vi "Acquisizione statica_1.vi"() -> ()   [LabVIEW 2017]
uses:
  <vilib>/Analysis/4window.llb/windowTd.ctl
  <vilib>/measure/maspectr.llb/Power Spectrum and PSD Export Mode.ctl
  <vilib>/DAQmx/read.llb/DAQmx Read (Analog 1D Wfm NChan NSamp).vi
  <vilib>/DAQmx/configure/timing.llb/DAQmx Timing (Sample Clock).vi
  <vilib>/DAQmx/miscellaneous.llb/DAQmx Fill In Error Info.vi
  <vilib>/measure/maspectr.llb/FFT Power Spectrum and PSD for N Chan.vi
  <vilib>/measure/maspectr.llb/FFT Spectrum (Mag-Phase) for N Chan.vi
  <vilib>/measure/maspectr.llb/Frequency Response Function (Mag-Phase) N-M.vi
  <vilib>/Waveform/WDTOps.llb/WDT Index Channel DBL.vi
  <vilib>/Waveform/WDTOps.llb/WDT Append Waveforms DBL.vi
  <vilib>/measure/NI_MAPro.lvlib
  <vilib>/Analysis/NI_AALPro.lvlib
panel:
  in  "temperatura":refnum<k21>
  out "Massa pesata":string
  out "iterazioni":i32
  out "errore":bool
  out "error out":errorcluster
  out "std dev":bool
  out "mean":bool
  out "sample":i32
  in  "std dev max":dbl=6e-07
  in  "mean/sample max":dbl=0.002
  out "mean/sample":dbl
  out "mean":dbl format="%0.2f"
  out "std dev/semple":dbl
  out "standard deviation":dbl format="%0.2f"
  in  "Massa":string="_"
  in  "secondi da salvare":i32=30
  in  "restart averaging (F)":bool
  in  "window":T1 items=["Rectangle"=0, "Hanning"=1, "Hamming"=2, "Blackman-Harris"=3, "Exact Blackman"=4, "Blackman"=5, "Flat Top"=6, "4 Term B-Harris "=7, "7 Term B-Harris"=8, "Low Sidelobe"=9, "Blackman Nuttall"=11, "Triangle"=30, "Bartlett-Hanning"=31, "Bohman"=32, "Parzen"=33, "Welch"=34, "Kaiser"=60, "Dolph-Chebyshev"=61, "Gaussian"=62]
  in  "averaging parameters":T2={"averaging mode"=enum."Vector averaging", "weighting mode"=enum."Linear", "number of averages"=1000}
  in  "Tab Control 2":enum32{"LC", "T", "FRF", "PSD", "FFT"}(tab)
  out "Load Cell":waveform(dbl)[](graph)
  out "Temperature":waveform(dbl)[](graph)
  out "Waveform Graph":cluster{"f0":dbl, "df":dbl, "magnitude":dbl[]}[](graph)
  out "Waveform Graph 2":cluster{"f0":dbl, "df":dbl, "magnitude":dbl[]}[](graph)
  out "Magnitude 2":cluster{"f0":dbl, "df":dbl, "magnitude":dbl[]}[](graph)
  out "Magnitude":cluster{"f0":dbl, "df":dbl, "magnitude":dbl[]}[](graph)
  in  "SAVE?":bool
  in  "export":path
  in  "stop":bool
  in  "acquisition":T3={"Fs"=2000.0, "group sample/s"=10, "generation task"="ModAnalEs"} {"Fs" format="%.2p"}
  # "0,002"
  # "x10^-3"
  # "x10^-6"
  # "6E-7"
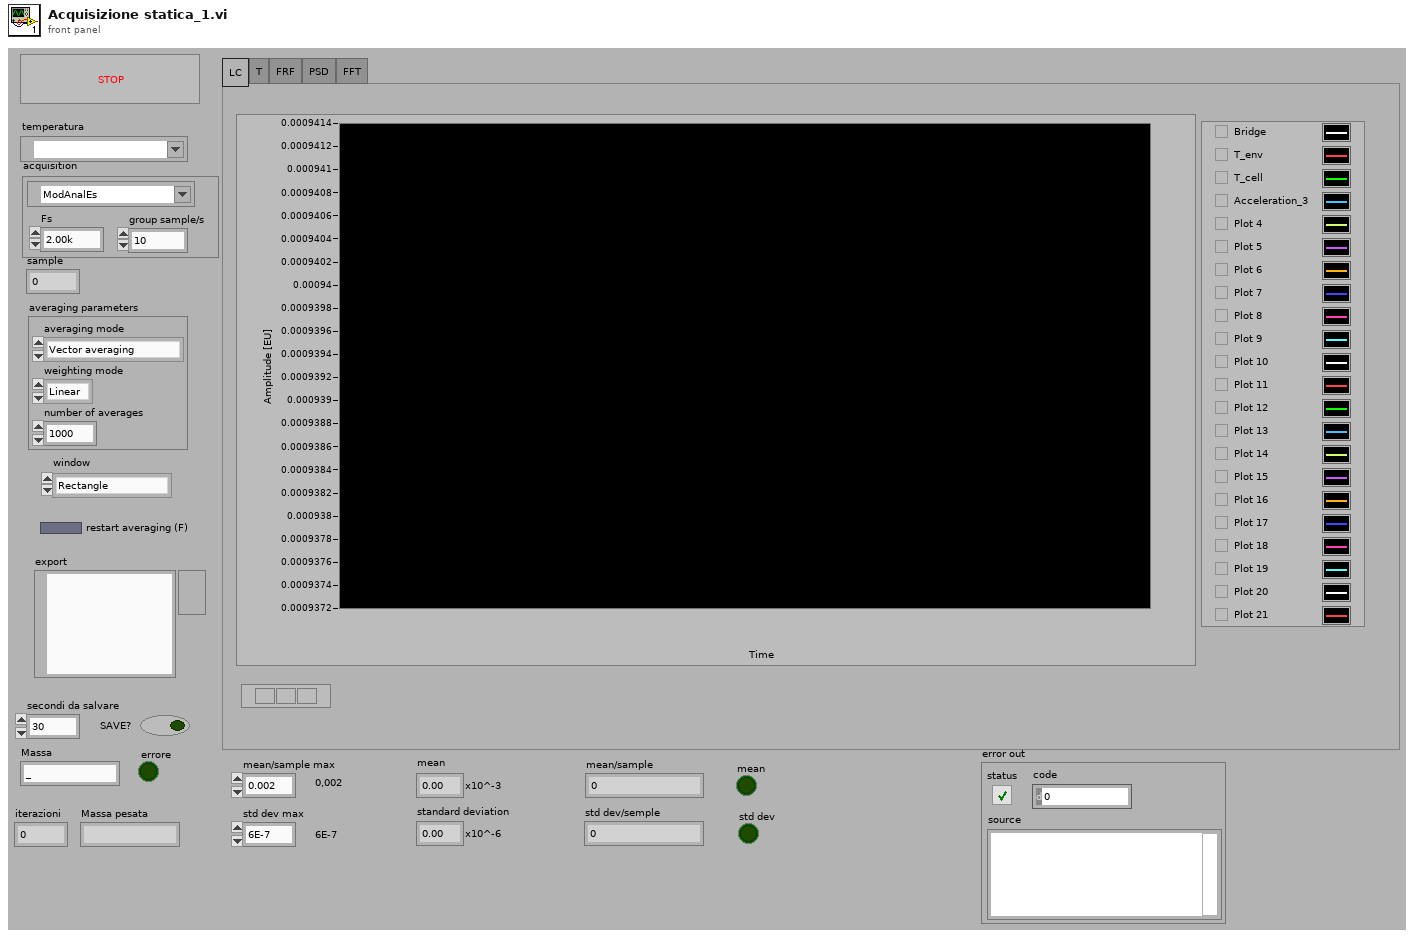
[diagram p1: front panel]
types:
  T1 = typedef "NI_AALPro.lvlib/windowTd.ctl" = u32
  T2 = cluster{"averaging mode":enum16{"No averaging", "Vector averaging", "RMS averaging", "Peak hold"}, "weighting mode":enum16{"Linear", "Exponential"}, "number of averages":u32}
  T3 = cluster{"Fs":dbl, "group sample/s":i32, "generation task":refnum<k21>}
  T4 = cluster{"dB On (F)":bool, "unwrap phase (F)":bool, "convert to degree (F)":bool}
  T5 = typedef "NI_MAPro.lvlib/Power Spectrum and PSD Export Mode.ctl" = u16
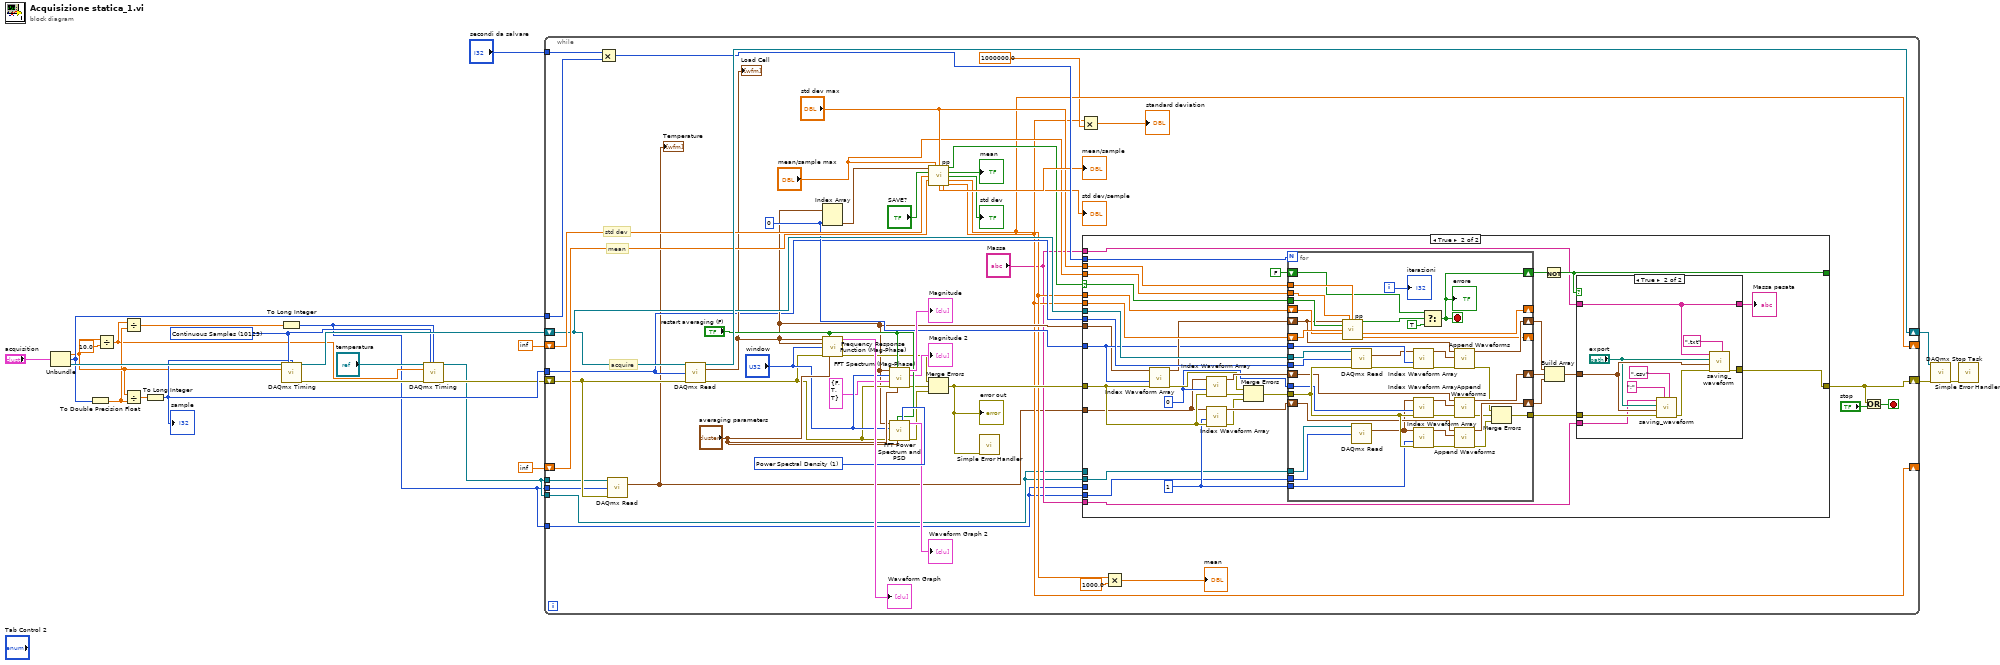
[diagram p0: block diagram]
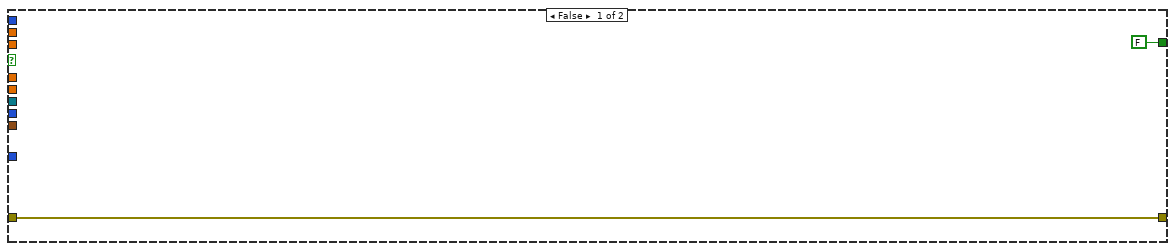
[diagram p2: hidden frame]
diagram:
  w11 = 10123 items=["Finite Samples"=10178, "Continuous Samples"=10123, "Hardware Timed Single Point"=12522] ("sample mode")
  n1 = Unbundle("acquisition") -> ("Fs"=w9:dbl, "group sample/s"=w13:i32, "generation task"=w20:refnum<k21>)
  n2 = To Double Precision Float(number=w13) -> (double precision float=w7:dbl)
  n3 = Divide(x=w9, y=10.0) -> (x/y=w3:dbl)
  n4 = Divide(x=w3, y=w7) -> (x/y=w6:dbl)
  n5 = Divide(x=w9, y=w7) -> (x/y=w16:dbl)
  n6 = To Long Integer(number=w16) -> (32bit integer=w10:i32)
  "sample" <- w10
  n7 = To Long Integer(number=w6) -> (32bit integer=w1:i32)
  n8 = call-poly <vilib>:"DAQmx Timing.vi"("task/channels in"=w20, "sample mode"=w11, "samples per channel"=w10, "rate"=w9) -> ("task out"=w19:refnum<k21>, "error out"=w5:errorcluster)  [unwired: 10 in]
  n9 = call-poly <vilib>:"DAQmx Timing.vi"("task/channels in"="temperatura", "sample mode"=w11, "samples per channel"=w1, "rate"=w3, "error in"=w5) -> ("task out"=w2:refnum<k21>, "error out"=w4:errorcluster)  [unwired: 9 in]
  n10 = while {
    shift-right: [w72] -> w22
    shift-left: w19 -> [w57]
    shift-right: [w60] -> w23
    shift-left: w4 -> [w29]
    tunnel: w13 -> [w56]
    shift-right: [w36] -> _
    shift-left: inf -> [w59]
    shift-right: [w32] -> _
    shift-left: inf -> [w58]
    tunnel: "secondi da salvare" -> [w54]
    tunnel: w10 -> [w37]
    tunnel: w2 -> [w27]
    tunnel: w1 -> [w28]
    tunnel: w2 -> [w25]
    tunnel: w1 -> [w24]
    stop <- w61 stop-if-true
    w40 = 0 ("REFERENCE CHANNEL")
    w70 = T5 1 items=["Power Spectrum", "Power Spectral Density"] ("export mode")
    # "mean"
    # "std dev"
    # "acquire"
    n11 = Multiply(x=w54, y=w56) -> (x*y=w55:i32)
    n12 = call-poly <vilib>:"DAQmx Read.vi"("task/channels in"=w27, "number of samples per channel"=w28, "error in"=w29) -> ("data"=w26:waveform(dbl)[])  [unwired: 10 in, 2 out]
    "Temperature" <- w26
    n13 = call-poly <vilib>:"DAQmx Read.vi"("task/channels in"=w57, "number of samples per channel"=w37, "error in"=w29) -> ("task out"=w72:refnum<k21>, "data"=w38:waveform(dbl)[], "error out"=w44:errorcluster)  [unwired: 10 in]
    "Load Cell" <- w38
    n14 = Index Array(array=w38, index #2=w40) -> (element #2=w53:waveform(dbl))  [unwired: 1 in, 1 out]
    n15 = call-poly <vilib>:"Frequency Response Function (Mag-Phase).vi"("time signals X"=w38, "restart averaging (F)"="restart averaging (F)", "time signals Y"=w38, "window"="window", "error in (no error)"=w44, "averaging parameters"="averaging parameters") -> ("magnitudes"=→"Waveform Graph":cluster{"f0":dbl, "df":dbl, "magnitude":dbl[]}[], "error out"=w41:errorcluster)  [unwired: 4 in, 4 out]
    n16 = call-poly <vilib>:"FFT Spectrum (Mag-Phase).vi"("averaging parameters"="averaging parameters", "restart averaging (F)"="restart averaging (F)", "error in (no error)"=w44, "view"=T4 {"dB On (F)"=FALSE, "unwrap phase (F)"=TRUE, "convert to degree (F)"=TRUE}, "window"="window", "time signals"=w38) -> ("error out"=w42:errorcluster, "phases"=→"Magnitude 2":cluster{"f0":dbl, "df":dbl, "phase":dbl[]}[], "magnitudes"=→"Magnitude":cluster{"f0":dbl, "df":dbl, "magnitude":dbl[]}[])  [unwired: 1 in, 2 out]
    n17 = call-poly <vilib>:"FFT Power Spectrum and PSD.vi"("export mode"=w70, "averaging parameters"="averaging parameters", "restart averaging (F)"="restart averaging (F)", "error in (no error)"=w44, "window"="window", "time signals"=w38) -> ("error out"=w43:errorcluster, "Power Spectrum / PSD"=→"Waveform Graph 2":cluster{"f0":dbl, "df":dbl, "magnitude":dbl[]}[])  [unwired: 2 in, 2 out]
    n18 = call "pp.vi"("Waveform"=w53, "mean/sample max"="mean/sample max", "std dev max"="std dev max", "SAVE?"="SAVE?", "prev std dev"=w59, "prev mean"=w58) -> ("out"=w49:bool, 6:"mean"=→"mean":bool, "std dev"=→"std dev":bool, 10:"mean"=w36:dbl, "std dev/semple"=→"std dev/semple":dbl, "mean/sample"=→"mean/sample":dbl, "standard deviation"=w32:dbl)  [unwired: 3 in]
    n19 = Merge Errors(w41, w42, w43) -> (w39:errorcluster)
    "error out" <- w39
    n20 = call <vilib>:"Simple Error Handler.vi"("error in (no error)"=w39) -> ()  [unwired: 4 in, 5 out]
    n21 = Multiply(x=w32, y=1000000.0) -> (x*y=→"standard deviation":dbl)
    n22 = case shown="True" w49 {
      selector: w49 -> [_ w102]
      tunnel: w39 -> [w74 w87]
      tunnel: [w74 w109] -> w60
      tunnel: w38 -> [_ w82]
      tunnel: w55 -> [_ w108]
      tunnel: w57 -> [_ w107]
      tunnel: w37 -> [_ w105]
      tunnel: w32 -> [_ w101]
      tunnel: w36 -> [_ w100]
      tunnel: "std dev max" -> [_ w99]
      tunnel: "mean/sample max" -> [_ w98]
      tunnel: [FALSE w95] -> _
      tunnel: w40 -> [_ w93]
      tunnel: "Massa" -> [_ w92]
      tunnel: "Massa" -> [_ w91]
      tunnel: w25 -> [_ _]
      tunnel: w24 -> [_ _]
      tunnel: w26 -> [_ w77]
      tunnel: w25 -> [_ w76]
      tunnel: w24 -> [_ w75]
      frame False {
      }
      frame True {
        w80 = 1 ("index")
        w81 = 0 ("index")
        n23 = call-poly <vilib>:"Index Waveform Array.vi"("error in (no error)"=w87, "index"=w93, "waveform array"=w82) -> ("error out"=w86:errorcluster, "waveform"=w94:waveform(dbl))  [unwired: 7 in]
        n24 = call-poly <vilib>:"Index Waveform Array.vi"("error in (no error)"=w87, "index"=w81, "waveform array"=w77) -> ("error out"=w85:errorcluster, "waveform"=w89:waveform(dbl))  [unwired: 7 in]
        n25 = call-poly <vilib>:"Index Waveform Array.vi"("error in (no error)"=w87, "index"=w80, "waveform array"=w77) -> ("error out"=w84:errorcluster, "waveform"=w88:waveform(dbl))  [unwired: 7 in]
        n26 = Merge Errors(w86, w85, w84) -> (w83:errorcluster)
        n27 = for {
          N: w108 -> [_]
          shift-right: [w148] -> w104
          shift-left: w94 -> [w131]
          tunnel: [w115] -> w106
          tunnel: w83 -> [w128]
          tunnel: w107 -> [w144]
          tunnel: w105 -> [w143]
          tunnel: w102 -> [w142]
          shift-right: [w138] -> _
          shift-left: w101 -> [w141]
          shift-right: [w139] -> _
          shift-left: w100 -> [w140]
          tunnel: w99 -> [w137]
          tunnel: w98 -> [w136]
          shift-right: [w129] -> w96
          shift-left: FALSE -> [w134]
          tunnel: w93 -> [w132]
          shift-right: [w124] -> w79
          shift-left: w89 -> [w126]
          shift-right: [w121] -> w78
          shift-left: w88 -> [w122]
          tunnel: w81 -> [w127]
          tunnel: w80 -> [w113]
          tunnel: w76 -> [w112]
          tunnel: w75 -> [w111]
          i -> [w130]
          stop <- w129 stop-if-true
          n28 = call "pp.vi"("Waveform"=w131, "mean/sample max"=w136, "std dev max"=w137, "SAVE?"=w142, "prev std dev"=w141, "prev mean"=w140) -> ("out"=w135:bool, "mean"=w139:dbl, "standard deviation"=w138:dbl)  [unwired: 3 in, 4 out]
          n29 = call-poly <vilib>:"DAQmx Read.vi"("task/channels in"=w144, "number of samples per channel"=w143, "error in"=w128) -> ("data"=w114:waveform(dbl)[], "error out"=w146:errorcluster)  [unwired: 10 in, 1 out]
          n30 = call-poly <vilib>:"DAQmx Read.vi"("task/channels in"=w112, "number of samples per channel"=w111) -> ("data"=w110:waveform(dbl)[])  [unwired: 11 in, 2 out]
          n31 = call-poly <vilib>:"Index Waveform Array.vi"("error in (no error)"=w146, "index"=w132, "waveform array"=w114) -> ("error out"=w145:errorcluster, "waveform"=w147:waveform(dbl))  [unwired: 7 in]
          n32 = call-poly <vilib>:"Index Waveform Array.vi"("error in (no error)"=w128, "index"=w127, "waveform array"=w110) -> ("error out"=w119:errorcluster, "waveform"=w125:waveform(dbl))  [unwired: 7 in]
          n33 = call-poly <vilib>:"Index Waveform Array.vi"("error in (no error)"=w128, "index"=w113, "waveform array"=w110) -> ("error out"=w120:errorcluster, "waveform"=w123:waveform(dbl))  [unwired: 7 in]
          n34 = Select(t=w134, s=w135, f=TRUE) -> (s? t:f=w129:bool)
          "errore" <- w129
          n35 = call-poly <vilib>:"Append Waveforms.vi"("error in (no error)"=w145, "waveform B"=w147, "waveform A"=w131) -> ("error out"=w116:errorcluster, "waveform out"=w148:waveform(dbl))  [unwired: 7 in]
          n36 = call-poly <vilib>:"Append Waveforms.vi"("error in (no error)"=w119, "waveform B"=w125, "waveform A"=w126) -> ("error out"=w117:errorcluster, "waveform out"=w124:waveform(dbl))  [unwired: 7 in]
          n37 = call-poly <vilib>:"Append Waveforms.vi"("error in (no error)"=w120, "waveform B"=w123, "waveform A"=w122) -> ("error out"=w118:errorcluster, "waveform out"=w121:waveform(dbl))  [unwired: 7 in]
          n38 = Merge Errors(w116, w117, w118) -> (w115:errorcluster)
          "iterazioni" <- w130
        }
        n39 = Not(x=w96) -> (.not. x?=w95:bool)
        n40 = Build Array(w104, w79, w78) -> (w103:waveform(dbl)[])
        n41 = case shown="True" w95 {
          tunnel: w103 -> [_ w158]
          tunnel: [w150 w154] -> w109
          tunnel: w106 -> [w150 w153]
          tunnel: w92 -> [w149 w151]
          tunnel: w91 -> [_ w152]
          tunnel: [w149 w151] -> w90
          frame False {
          }
          frame True {
            n42 = call "saving_waveform.vi"("extension"=".csv", "delimiter (Tab)"=";", "error in (no error)"=w153, "Array"=w158, "directory"="export", "Massa"=w152) -> ("error out"=w155:errorcluster)  [unwired: 5 in]
            n43 = call "saving_waveform.vi"("extension"=".txt", "error in (no error)"=w155, "Array"=w158, "directory"="export", "Massa"=w151) -> ("error out"=w154:errorcluster)  [unwired: 6 in]
          }
        }
        "Massa pesata" <- w90
      }
    }
    n44 = Multiply(x=w36, y=1000.0) -> (x*y=→"mean":dbl)
    n45 = Or(x=w60, y="stop") -> (x .or. y?=w61:bool)
  }
  n46 = call <vilib>:"DAQmx Stop Task.vi"("task/channels in"=w22, "error in"=w23) -> ("error out"=w18:errorcluster)  [unwired: 12 in, 1 out]
  n47 = call <vilib>:"Simple Error Handler.vi"("error in (no error)"=w18) -> ()  [unwired: 4 in, 5 out]
